vi "Főképernyő UI engedélyezés.vi"(8 "Error In":errorcluster, 9 "Jogosultságok array":T1[](array[typedef]), 10 "Felhasználói szint":string, 11 "UI Data":T2) -> (0 "Error Out":errorcluster, 2 "Felhasználói szint ki":string, 3 "UI Data out":T2)   [LabVIEW 2014]
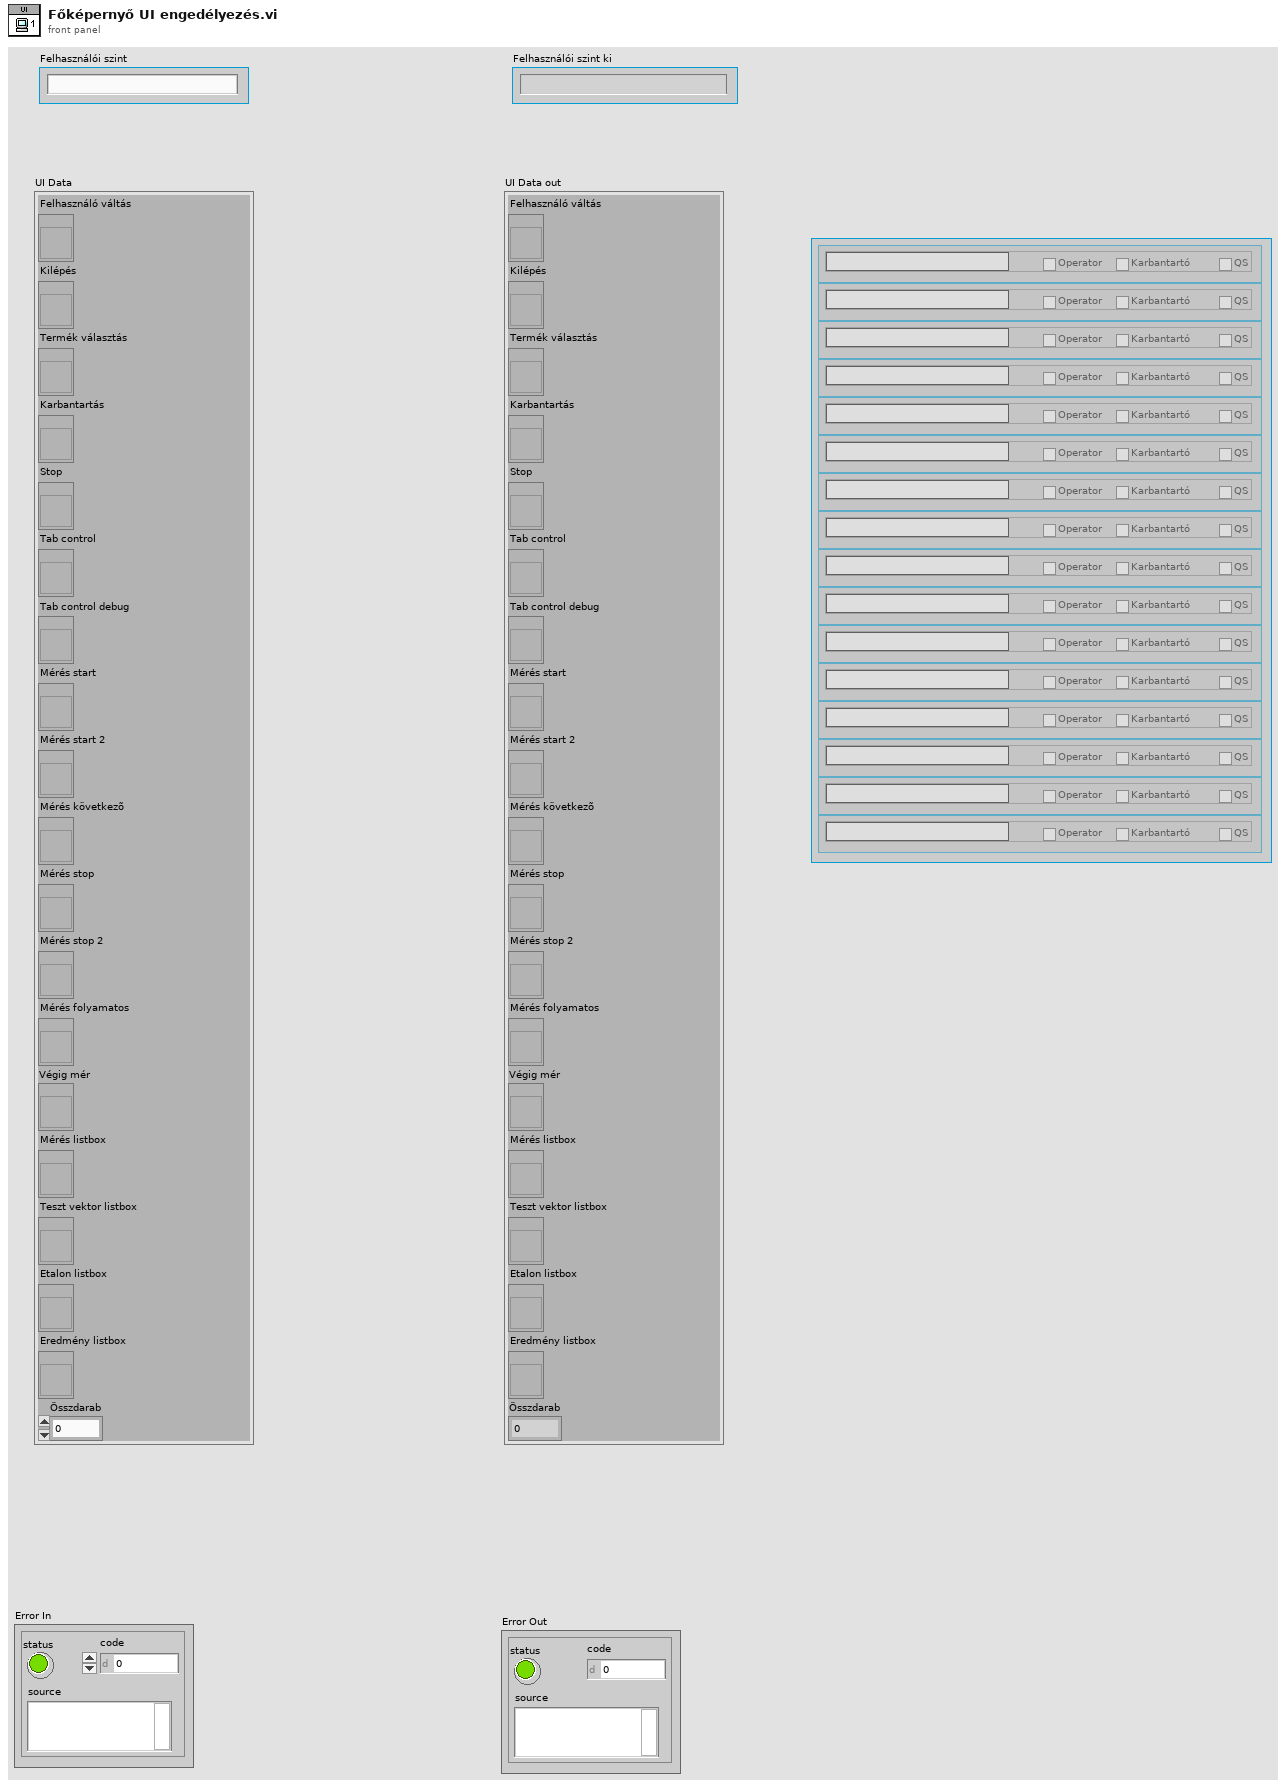
[diagram p1: front panel]
types:
  T1 = typedef "Tab jogosultság.ctl" = cluster{"Tab Name":string, "Operator":bool, "Karbantartó":bool, "QS":bool}
  T2 = typedef "Fõképernyõ references.ctl" = cluster{"Felhasználó váltás":refnum<vi>, "Kilépés":refnum<vi>, "Termék választás":refnum<vi>, "Karbantartás":refnum<vi>, "Stop":refnum<vi>, "Tab control":refnum<vi>, "Tab control debug":refnum<vi>, "Mérés start":refnum<vi>, "Mérés start 2":refnum<vi>, "Mérés következõ":refnum<vi>, "Mérés stop":refnum<vi>, "Mérés stop 2":refnum<vi>, "Mérés folyamatos":refnum<vi>, "Végig mér":refnum<vi>, "Mérés listbox":refnum<vi>, "Teszt vektor listbox":refnum<vi>, "Etalon listbox":refnum<vi>, "Eredmény listbox":refnum<vi>, "Összdarab":i64}
  T3 = enum8{"Enabled", "Disabled", "Disabled and Grayed Out"}
  T4 = enum32{"Page Enabled", "Page Disabled", "Page Disabled & Grayed"}
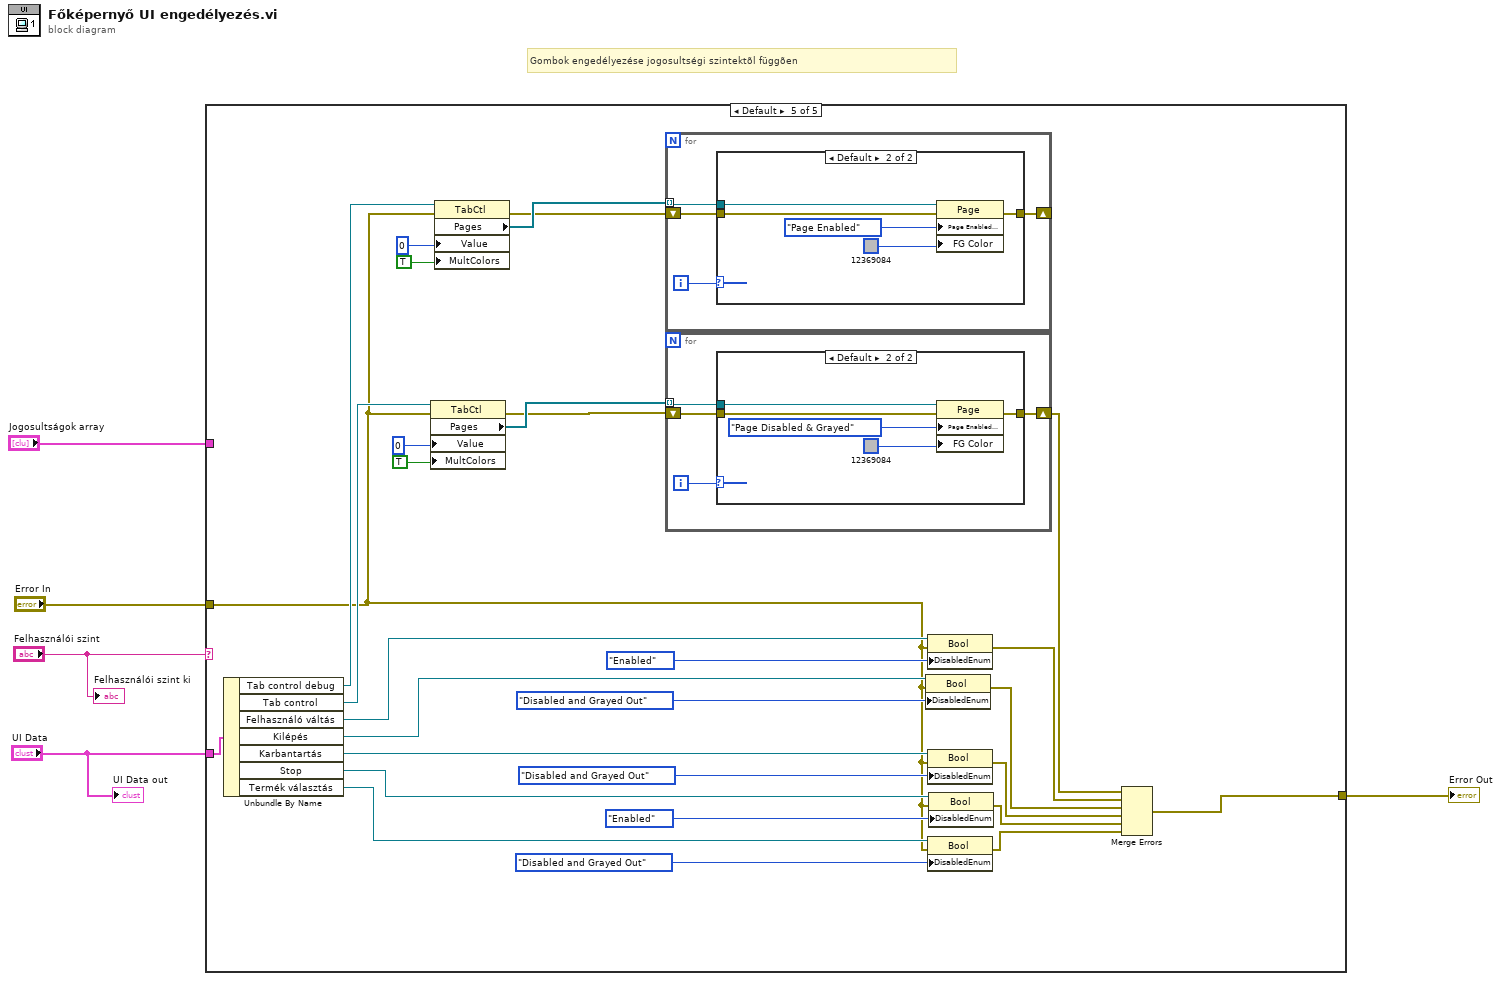
[diagram p0: block diagram]
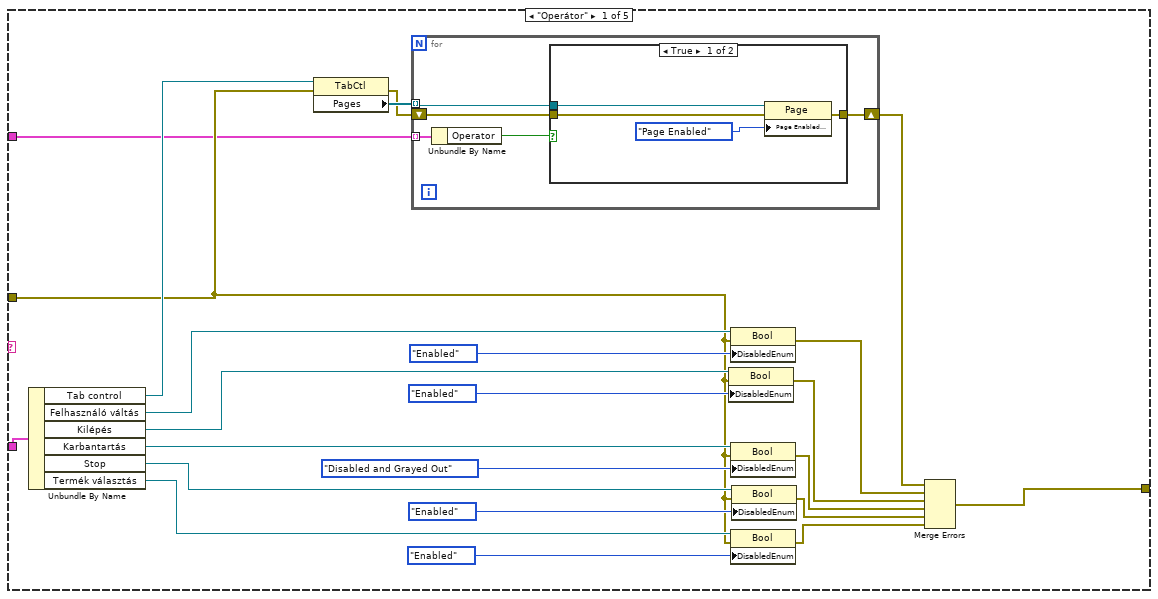
[diagram p2: hidden frame]
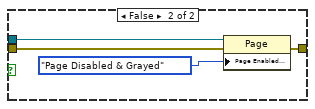
[diagram p3: hidden frame]
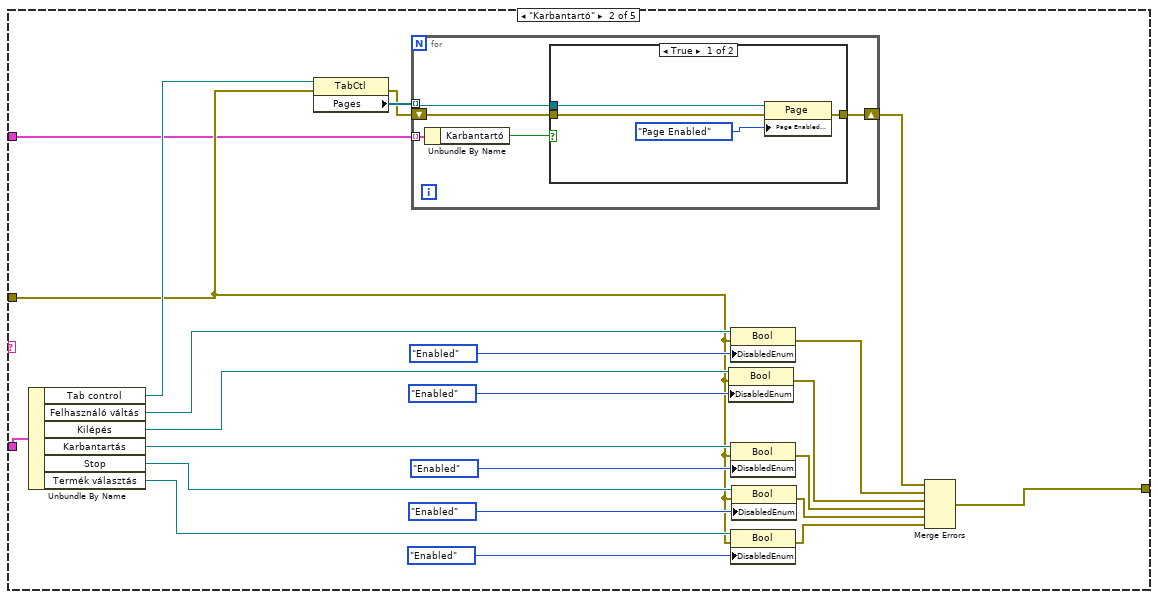
[diagram p4: hidden frame]
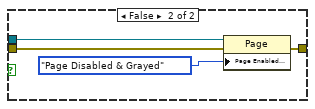
[diagram p5: hidden frame]
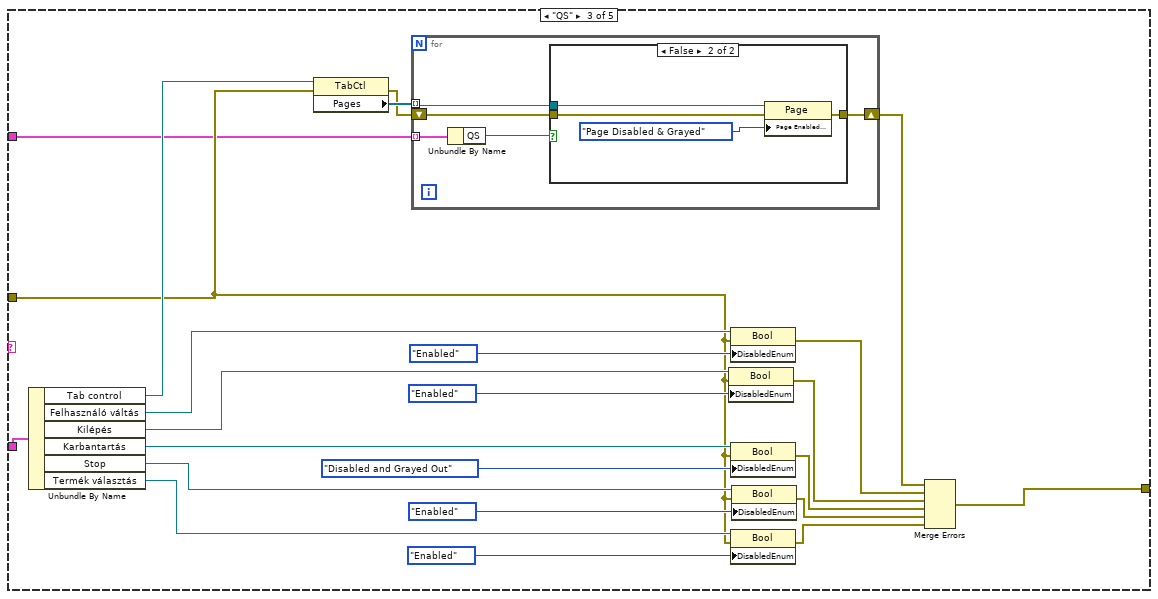
[diagram p6: hidden frame]
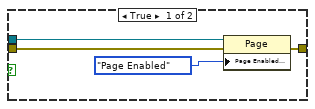
[diagram p7: hidden frame]
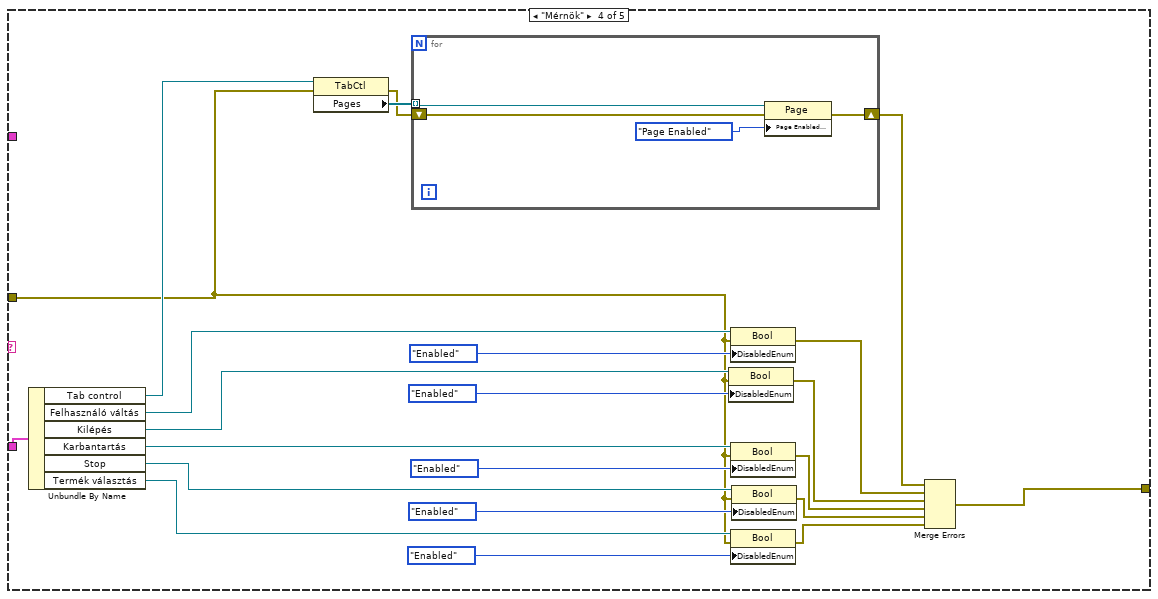
[diagram p8: hidden frame]
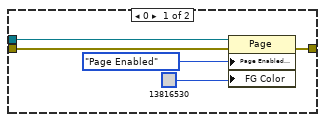
[diagram p9: hidden frame]
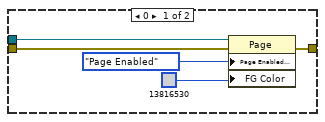
[diagram p10: hidden frame]
diagram:
  # "Gombok engedélyezése jogosultségi szintektõl függõen"
  n1 = case shown="Default" "Felhasználói szint" {
    tunnel: "Error In" -> [w8 w44 w80 w115 w143]
    tunnel: [w22 w58 w94 w129 w162] -> w4
    tunnel: "UI Data" -> [w21 w57 w93 w128 w161]
    tunnel: "Jogosultságok array" -> [w6 w42 w78 _ _]
    frame "Operátor" {
      n2 = Unbundle By Name(w21) -> ("Tab control"=w20:refnum<vi>, "Felhasználó váltás"=w19:refnum<vi>, "Kilépés"=w18:refnum<vi>, "Karbantartás"=w17:refnum<vi>, "Stop"=w14:refnum<vi>, "Termék választás"=w13:refnum<vi>)
      n3 = property on="Property Node" class="TabCtl"(reference=w20, error in=w8) -> (error out=w9:errorcluster, "Pages"=w10:refnum<vi>[])  [unwired: 1 out]
      n4 = for {
        shift-right: [w33] -> w7
        shift-left: w9 -> [w32]
        tunnel: w10 -> [w31] mode=indexing
        tunnel: w6 -> [w30] mode=indexing
        n5 = Unbundle By Name(w30) -> ("Operator"=w29:bool)
        n6 = case shown="True" w29 {
          tunnel: [w37 w41] -> w33
          tunnel: w32 -> [w36 w40]
          tunnel: w31 -> [w35 w39]
          frame True {
            n7 = property class="Page"(reference=w35, error in=w36, "Page Enabled State"=T4."Page Enabled") -> (error out=w37:errorcluster)  [unwired: 1 out]
          }
          frame False {
            n8 = property class="Page"(reference=w39, error in=w40, "Page Enabled State"=T4."Page Disabled & Grayed") -> (error out=w41:errorcluster)  [unwired: 1 out]
          }
        }
      }
      n9 = property on="Property Node" class="Bool"(reference=w18, error in=w8, "DisabledEnum"=T3."Enabled" ("Disabled")) -> (error out=w25:errorcluster)  [unwired: 1 out]
      n10 = property on="Property Node" class="Bool"(reference=w19, error in=w8, "DisabledEnum"=T3."Enabled" ("Disabled")) -> (error out=w26:errorcluster)  [unwired: 1 out]
      n11 = property on="Property Node" class="Bool"(reference=w17, error in=w8, "DisabledEnum"=T3."Disabled and Grayed Out" ("Disabled")) -> (error out=w24:errorcluster)  [unwired: 1 out]
      n12 = property on="Property Node" class="Bool"(reference=w13, error in=w8, "DisabledEnum"=T3."Enabled" ("Disabled")) -> (error out=w11:errorcluster)  [unwired: 1 out]
      n13 = property on="Property Node" class="Bool"(reference=w14, error in=w8, "DisabledEnum"=T3."Enabled" ("Disabled")) -> (error out=w23:errorcluster)  [unwired: 1 out]
      n14 = Merge Errors(w7, w26, w25, w24, w23, w11) -> (w22:errorcluster)
    }
    frame "Karbantartó" {
      n15 = Unbundle By Name(w57) -> ("Tab control"=w56:refnum<vi>, "Felhasználó váltás"=w55:refnum<vi>, "Kilépés"=w54:refnum<vi>, "Karbantartás"=w53:refnum<vi>, "Stop"=w50:refnum<vi>, "Termék választás"=w49:refnum<vi>)
      n16 = property on="Property Node" class="TabCtl"(reference=w56, error in=w44) -> (error out=w45:errorcluster, "Pages"=w46:refnum<vi>[])  [unwired: 1 out]
      n17 = for {
        shift-right: [w69] -> w43
        shift-left: w45 -> [w68]
        tunnel: w46 -> [w67] mode=indexing
        tunnel: w42 -> [w66] mode=indexing
        n18 = Unbundle By Name(w66) -> ("Karbantartó"=w65:bool)
        n19 = case shown="True" w65 {
          tunnel: [w73 w77] -> w69
          tunnel: w68 -> [w72 w76]
          tunnel: w67 -> [w71 w75]
          frame True {
            n20 = property class="Page"(reference=w71, error in=w72, "Page Enabled State"=T4."Page Enabled") -> (error out=w73:errorcluster)  [unwired: 1 out]
          }
          frame False {
            n21 = property class="Page"(reference=w75, error in=w76, "Page Enabled State"=T4."Page Disabled & Grayed") -> (error out=w77:errorcluster)  [unwired: 1 out]
          }
        }
      }
      n22 = property on="Property Node" class="Bool"(reference=w54, error in=w44, "DisabledEnum"=T3."Enabled" ("Disabled")) -> (error out=w61:errorcluster)  [unwired: 1 out]
      n23 = property on="Property Node" class="Bool"(reference=w55, error in=w44, "DisabledEnum"=T3."Enabled" ("Disabled")) -> (error out=w62:errorcluster)  [unwired: 1 out]
      n24 = property on="Property Node" class="Bool"(reference=w53, error in=w44, "DisabledEnum"=T3."Enabled" ("Disabled")) -> (error out=w60:errorcluster)  [unwired: 1 out]
      n25 = property on="Property Node" class="Bool"(reference=w49, error in=w44, "DisabledEnum"=T3."Enabled" ("Disabled")) -> (error out=w47:errorcluster)  [unwired: 1 out]
      n26 = property on="Property Node" class="Bool"(reference=w50, error in=w44, "DisabledEnum"=T3."Enabled" ("Disabled")) -> (error out=w59:errorcluster)  [unwired: 1 out]
      n27 = Merge Errors(w43, w62, w61, w60, w59, w47) -> (w58:errorcluster)
    }
    frame "QS" {
      n28 = Unbundle By Name(w93) -> ("Tab control"=w92:refnum<vi>, "Felhasználó váltás"=w91:refnum<vi>, "Kilépés"=w90:refnum<vi>, "Karbantartás"=w89:refnum<vi>, "Stop"=w86:refnum<vi>, "Termék választás"=w85:refnum<vi>)
      n29 = property on="Property Node" class="TabCtl"(reference=w92, error in=w80) -> (error out=w81:errorcluster, "Pages"=w82:refnum<vi>[])  [unwired: 1 out]
      n30 = for {
        shift-right: [w105] -> w79
        shift-left: w81 -> [w104]
        tunnel: w82 -> [w103] mode=indexing
        tunnel: w78 -> [w102] mode=indexing
        n31 = Unbundle By Name(w102) -> ("QS"=w101:bool)
        n32 = case shown="False" w101 {
          tunnel: [w109 w113] -> w105
          tunnel: w104 -> [w108 w112]
          tunnel: w103 -> [w107 w111]
          frame True {
            n33 = property class="Page"(reference=w107, error in=w108, "Page Enabled State"=T4."Page Enabled") -> (error out=w109:errorcluster)  [unwired: 1 out]
          }
          frame False {
            n34 = property class="Page"(reference=w111, error in=w112, "Page Enabled State"=T4."Page Disabled & Grayed") -> (error out=w113:errorcluster)  [unwired: 1 out]
          }
        }
      }
      n35 = property on="Property Node" class="Bool"(reference=w90, error in=w80, "DisabledEnum"=T3."Enabled" ("Disabled")) -> (error out=w97:errorcluster)  [unwired: 1 out]
      n36 = property on="Property Node" class="Bool"(reference=w91, error in=w80, "DisabledEnum"=T3."Enabled" ("Disabled")) -> (error out=w98:errorcluster)  [unwired: 1 out]
      n37 = property on="Property Node" class="Bool"(reference=w89, error in=w80, "DisabledEnum"=T3."Disabled and Grayed Out" ("Disabled")) -> (error out=w96:errorcluster)  [unwired: 1 out]
      n38 = property on="Property Node" class="Bool"(reference=w85, error in=w80, "DisabledEnum"=T3."Enabled" ("Disabled")) -> (error out=w83:errorcluster)  [unwired: 1 out]
      n39 = property on="Property Node" class="Bool"(reference=w86, error in=w80, "DisabledEnum"=T3."Enabled" ("Disabled")) -> (error out=w95:errorcluster)  [unwired: 1 out]
      n40 = Merge Errors(w79, w98, w97, w96, w95, w83) -> (w94:errorcluster)
    }
    frame "Mérnök" {
      n41 = Unbundle By Name(w128) -> ("Tab control"=w127:refnum<vi>, "Felhasználó váltás"=w126:refnum<vi>, "Kilépés"=w125:refnum<vi>, "Karbantartás"=w124:refnum<vi>, "Stop"=w121:refnum<vi>, "Termék választás"=w120:refnum<vi>)
      n42 = property on="Property Node" class="TabCtl"(reference=w127, error in=w115) -> (error out=w116:errorcluster, "Pages"=w117:refnum<vi>[])  [unwired: 1 out]
      n43 = for {
        shift-right: [w139] -> w114
        shift-left: w116 -> [w138]
        tunnel: w117 -> [w137] mode=indexing
        n44 = property class="Page"(reference=w137, error in=w138, "Page Enabled State"=T4."Page Enabled") -> (error out=w139:errorcluster)  [unwired: 1 out]
      }
      n45 = property on="Property Node" class="Bool"(reference=w125, error in=w115, "DisabledEnum"=T3."Enabled" ("Disabled")) -> (error out=w132:errorcluster)  [unwired: 1 out]
      n46 = property on="Property Node" class="Bool"(reference=w126, error in=w115, "DisabledEnum"=T3."Enabled" ("Disabled")) -> (error out=w133:errorcluster)  [unwired: 1 out]
      n47 = property on="Property Node" class="Bool"(reference=w124, error in=w115, "DisabledEnum"=T3."Enabled" ("Disabled")) -> (error out=w131:errorcluster)  [unwired: 1 out]
      n48 = property on="Property Node" class="Bool"(reference=w120, error in=w115, "DisabledEnum"=T3."Enabled" ("Disabled")) -> (error out=w118:errorcluster)  [unwired: 1 out]
      n49 = property on="Property Node" class="Bool"(reference=w121, error in=w115, "DisabledEnum"=T3."Enabled" ("Disabled")) -> (error out=w130:errorcluster)  [unwired: 1 out]
      n50 = Merge Errors(w114, w133, w132, w131, w130, w118) -> (w129:errorcluster)
    }
    frame Default {
      n51 = Unbundle By Name(w161) -> ("Tab control debug"=w144:refnum<vi>, "Tab control"=w147:refnum<vi>, "Felhasználó váltás"=w160:refnum<vi>, "Kilépés"=w159:refnum<vi>, "Karbantartás"=w158:refnum<vi>, "Stop"=w155:refnum<vi>, "Termék választás"=w154:refnum<vi>)
      n52 = property on="Property Node" class="TabCtl"(reference=w147, error in=w143, "Value"=0, "MultColors"=TRUE ("Allow Multiple Colors")) -> (error out=w141:errorcluster, "Pages"=w150:refnum<vi>[])  [unwired: 1 out]
      n53 = property on="Property Node" class="TabCtl"(reference=w144, error in=w143, "Value"=0, "MultColors"=TRUE ("Allow Multiple Colors")) -> (error out=w140:errorcluster, "Pages"=w142:refnum<vi>[])  [unwired: 1 out]
      n54 = for {
        shift-right: [w172] -> _
        shift-left: w140 -> [w171]
        tunnel: w142 -> [w170] mode=indexing
        i -> [w169]
        n55 = case shown="Default" w169 {
          tunnel: [w177 w182] -> w172
          tunnel: w171 -> [w176 w181]
          tunnel: w170 -> [w175 w180]
          frame 0 {
            n56 = property class="Page"(reference=w175, error in=w176, "Page Enabled State"=T4."Page Enabled", "FG Color"=u32 13816530) -> (error out=w177:errorcluster)  [unwired: 1 out]
          }
          frame Default {
            n57 = property class="Page"(reference=w180, error in=w181, "Page Enabled State"=T4."Page Enabled", "FG Color"=u32 12369084) -> (error out=w182:errorcluster)  [unwired: 1 out]
          }
        }
      }
      n58 = for {
        shift-right: [w186] -> w148
        shift-left: w141 -> [w185]
        tunnel: w150 -> [w184] mode=indexing
        i -> [w183]
        n59 = case shown="Default" w183 {
          tunnel: [w191 w196] -> w186
          tunnel: w185 -> [w190 w195]
          tunnel: w184 -> [w189 w194]
          frame 0 {
            n60 = property class="Page"(reference=w189, error in=w190, "Page Enabled State"=T4."Page Enabled", "FG Color"=u32 13816530) -> (error out=w191:errorcluster)  [unwired: 1 out]
          }
          frame Default {
            n61 = property class="Page"(reference=w194, error in=w195, "Page Enabled State"=T4."Page Disabled & Grayed", "FG Color"=u32 12369084) -> (error out=w196:errorcluster)  [unwired: 1 out]
          }
        }
      }
      n62 = property on="Property Node" class="Bool"(reference=w159, error in=w143, "DisabledEnum"=T3."Disabled and Grayed Out" ("Disabled")) -> (error out=w165:errorcluster)  [unwired: 1 out]
      n63 = property on="Property Node" class="Bool"(reference=w160, error in=w143, "DisabledEnum"=T3."Enabled" ("Disabled")) -> (error out=w166:errorcluster)  [unwired: 1 out]
      n64 = property on="Property Node" class="Bool"(reference=w158, error in=w143, "DisabledEnum"=T3."Disabled and Grayed Out" ("Disabled")) -> (error out=w164:errorcluster)  [unwired: 1 out]
      n65 = property on="Property Node" class="Bool"(reference=w154, error in=w143, "DisabledEnum"=T3."Disabled and Grayed Out" ("Disabled")) -> (error out=w152:errorcluster)  [unwired: 1 out]
      n66 = property on="Property Node" class="Bool"(reference=w155, error in=w143, "DisabledEnum"=T3."Enabled" ("Disabled")) -> (error out=w163:errorcluster)  [unwired: 1 out]
      n67 = Merge Errors(w148, w166, w165, w164, w163, w152) -> (w162:errorcluster)
    }
  }
  "Error Out" <- w4
  "UI Data out" <- "UI Data"
  "Felhasználói szint ki" <- "Felhasználói szint"
